vi "DRC91GetSetPoint.vi"(0 "VISA Rsrc":refnum<visa-resource-name>="GPIB0::12::INSTR", 11 "error in (no error)":errorcluster) -> (4 "SetPoint":dbl, 6 "Units":string, 15 "error out":errorcluster)   [LabVIEW 2010]
doc: "Ce VI lit les paramètres limites de contrôle et ceux de stabilisation du contrôleur."
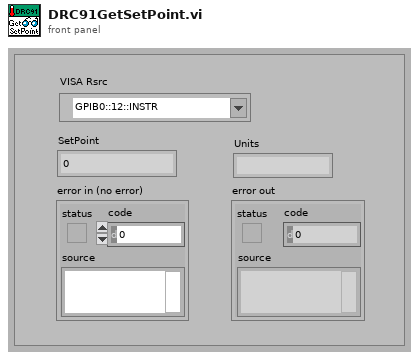
[diagram p1: front panel]
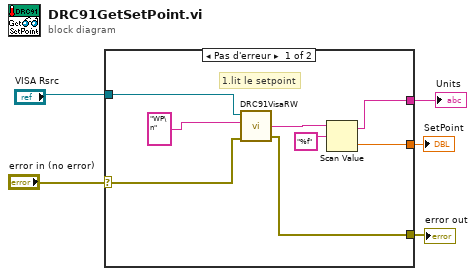
[diagram p0: block diagram]
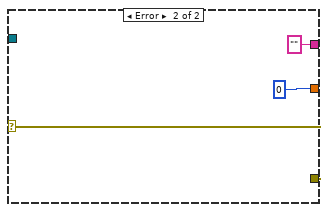
[diagram p2: hidden frame]
diagram:
  n1 = case shown="Pas d'erreur" "error in (no error)" {
    selector: "error in (no error)" -> [w12 w16]
    tunnel: "VISA Rsrc" -> [w13 _]
    tunnel: [w11 w16] -> w4
    tunnel: [w9 u32 0] -> w2
    tunnel: [w6 "" ("ChaineRep")] -> w1
    frame No Error {
      # "1.lit le setpoint"
      n2 = call <userlib>:"DRC91VisaRW.vi"("error in (no error)"=w12, "ChaineCom"="WP\n", "VISA Rsrc"=w13) -> ("error out"=w11:errorcluster, "ChaineRep"=w10:string)  [unwired: 4 in, 2 out]
      n3 = Scan Value(string=w10, format string="%f") -> (output string=w6:string, value=w9:dbl)  [unwired: 1 in]
    }
    frame Error {
    }
  }
  "error out" <- w4
  "SetPoint" <- w2
  "Units" <- w1
